vi "Parse-attribute.vi"(8 "error in (no error)":errorcluster, 10 "String in":string, 11 "Transform in":refnum<class "Transform.lvclass">) -> (0 "error out":errorcluster, 1 "Valid attribute?":bool, 2 "Remaining string":string, 3 "Transform out":refnum<class "Transform.lvclass">)   [LabVIEW 2013, in "HardwareCharacterization.lvlib" / "Transform.lvclass"]
uses:
  Transform.lvclass
  Attributes.ctl
  Attribute-ID.ctl
  Attribute-XML.lvclass/Attribute-XML.ctl
  ID.lvclass/ID.ctl
  Transform.lvclass/Transform.ctl
  Write Attribute.vi
  Write ID-attribute.vi
  Write Transformation matrix.vi
  Attribute-XML.lvclass
  ID.lvclass
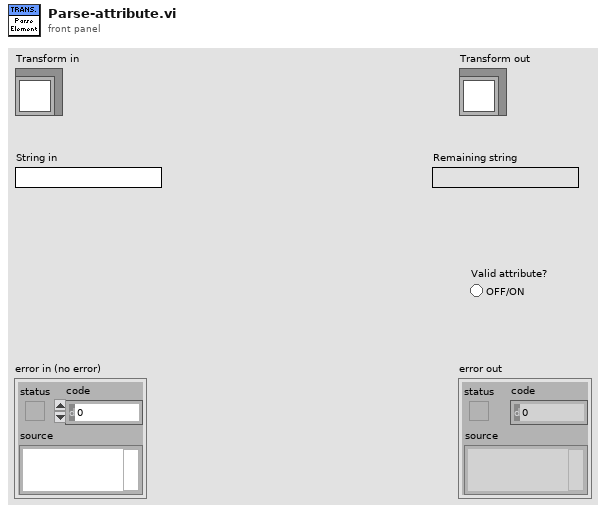
[diagram p1: front panel]
types:
  T1 = typedef "HardwareCharacterization.lvlib/ID.lvclass/Attribute-ID.ctl" = enum16{"FieldOffset", "TransformEnable", "Transform", "Units", "XYCalFactor", "EnableLaser", "JumpDelay", "MarkDelay", "PolyDelay", "LaserOnDelay", "LaserOffDelay", "JumpSpeed", "MarkSpeed", "LaserPowerDelay", "LaserEnableDelay", "LaserPower", "Offset"}
  T2 = typedef "HardwareCharacterization.lvlib/Attribute-XML.lvclass/Attributes.ctl" = enum16{"id"}
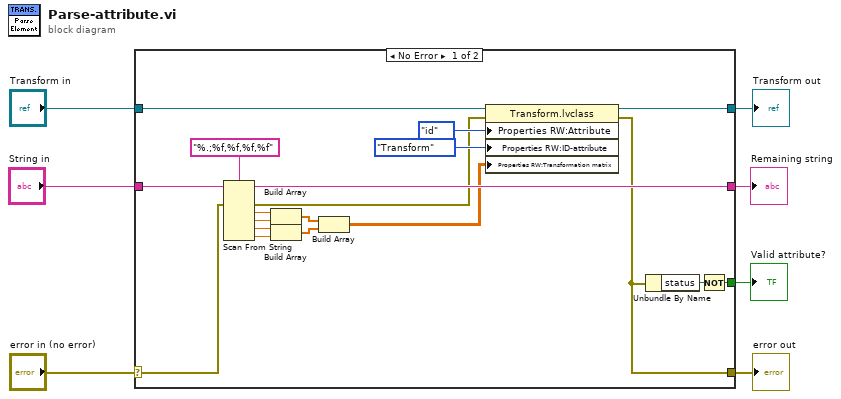
[diagram p0: block diagram]
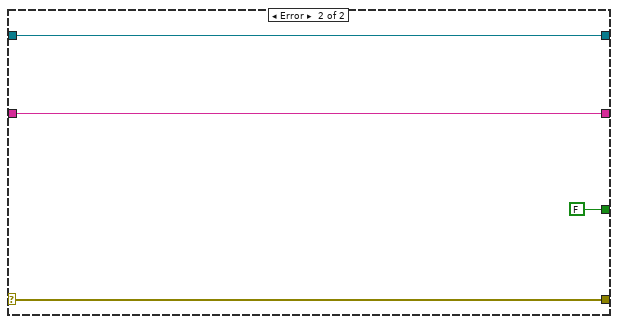
[diagram p2: hidden frame]
diagram:
  n1 = case shown="No Error" "error in (no error)" {
    selector: "error in (no error)" -> [w21 w30]
    tunnel: [w12 w30] -> w6
    tunnel: [w13 w29] -> w4
    tunnel: "Transform in" -> [w14 w29]
    tunnel: "String in" -> [w24 w28]
    tunnel: [w23 w28] -> w2
    tunnel: [w22 FALSE] -> w1
    frame No Error {
      n2 = Scan From String(format string="%.;%f,%f,%f,%f", input string=w24, error in=w21) -> (remaining string=w23:string, error out=w8:errorcluster, output 1=w19:dbl, output 2=w20:dbl, output 3=w18:dbl, output 4=w17:dbl)  [unwired: 5 in, 1 out]
      n3 = Build Array(w19, w20) -> (w16:dbl[])
      n4 = Build Array(w18, w17) -> (w15:dbl[])
      n5 = Build Array(w16, w15) -> (w9:dbl[][])
      n6 = property class="Transform.lvclass"(reference=w14, error in=w8, "Properties RW:Attribute"=Attributes."id" ("Attribute"), "Properties RW:ID-attribute"=Attribute-ID."Transform" ("ID-attribute"), "Properties RW:Transformation matrix"=w9) -> (reference out=w13:refnum<class "Transform.lvclass">, error out=w12:errorcluster)
      n7 = Unbundle By Name(w12) -> ("status"=w25:bool)
      n8 = Not(x=w25) -> (.not. x?=w22:bool)
    }
    frame Error {
    }
  }
  "error out" <- w6
  "Transform out" <- w4
  "Remaining string" <- w2
  "Valid attribute?" <- w1
